vi "translate_in.vi"(5 "InnerBlock type":refnum<class "InnerBlock.lvclass">, 8 "error in (no error)":errorcluster, 11 "OuterBlock":refnum<class "Block.lvclass">) -> (0 "error out":errorcluster, 3 "InnerBlock":refnum<class "InnerBlock.lvclass">)   [LabVIEW 2020, in "variant.lvlib" / "InnerBlock.lvclass"]
uses:
  InnerBlock.lvclass
  C:/projects/OpenG-Variant-Data-Library/source/library/Range/Block.lvclass
  Range/Block.lvclass
  InnerBlock.lvclass/InnerBlock.ctl
panel:
  in  "size":i32
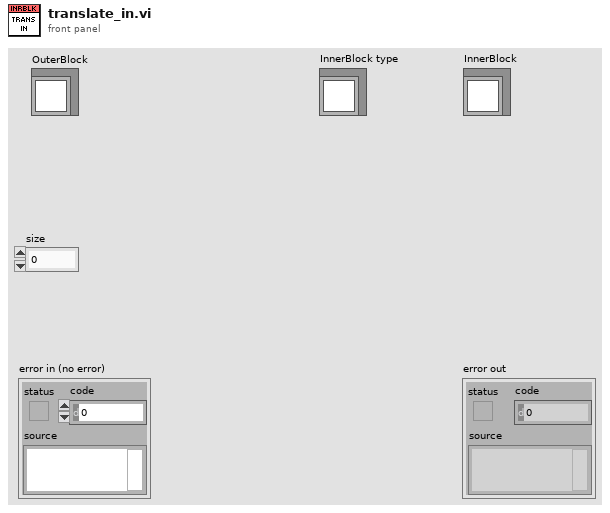
[diagram p1: front panel]
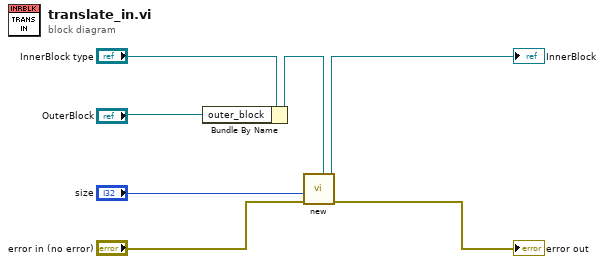
[diagram p0: block diagram]
diagram:
  n1 = Bundle By Name(cluster="InnerBlock type", "outer_block"="OuterBlock") -> (w5:refnum<class "InnerBlock.lvclass">)
  n2 = call "new.vi"("Range in"=w5, "error in (no error)"="error in (no error)", "size"="size") -> ("error out"=→"error out":errorcluster, "Range out"=→"InnerBlock":refnum<class "InnerBlock.lvclass">)  [unwired: 7 in]
